vi "SetTemp.vi"(8 "error in (no error)":errorcluster, 9 "Humid":dbl, 10 "Temp":dbl, 11 "Execute":refnum<class "Execute.lvclass">) -> (0 "error out":errorcluster, 3 "Execute":refnum<class "Execute.lvclass">)   [LabVIEW 2018, in "QMH_Class.lvlib" / "TestManager.lvlib" / "Execute.lvclass"]
uses:
  Execute.lvclass
  Execute.lvclass/Execute.ctl
  Device/TempChamber/TempChamber Interface/TempChamber Interface.lvclass
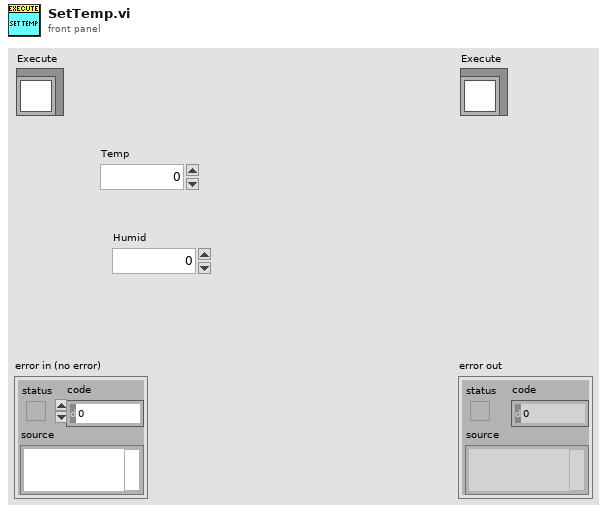
[diagram p1: front panel]
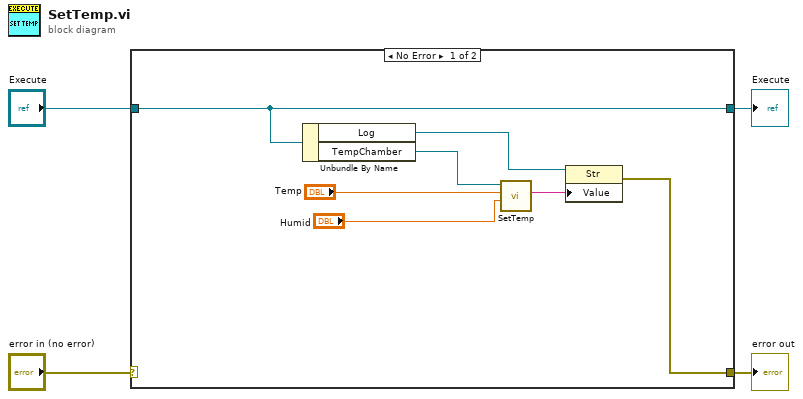
[diagram p0: block diagram]
diagram:
  n1 = case shown="No Error" "error in (no error)" {
    selector: "error in (no error)" -> [_ w13]
    tunnel: [w9 w13] -> w3
    tunnel: [w11 w12] -> w1
    tunnel: "Execute" -> [w11 w12]
    frame No Error {
      n2 = Unbundle By Name(w11) -> ("Log"=w10:refnum<vi>, "TempChamber"=w8:refnum<class "TempChamber Interface.lvclass">)
      n3 = call-dynamic "SetTemp.vi"("Humid"="Humid", "Temp"="Temp", "TempChamber Interface in"=w8) -> ("Fb"=w7:string)  [unwired: 6 in, 2 out]
      n4 = property class="Str"(reference=w10, "Value"=w7) -> (error out=w9:errorcluster)  [unwired: 1 in, 1 out]
    }
    frame Error {
    }
  }
  "error out" <- w3
  "Execute" <- w1
